vi "ATM_CLD.vi"(4 "Enter":bool, 6 "User Input":string, 7 "Card Simulator":bool, 10 "Right Buttons":T3, 11 "Left Buttons":T4) -> (0 "error out":errorcluster, 3 "ATM Messages":string, 8 "Right Menu":T1, 9 "Left Menu":T2)   [LabVIEW 2018]
doc: "ATM Version 1.0: final solution. Extensive documentation and VI appearance added"
uses:
  Controls/ATMStates.ctl
  Controls/Customer.ctl
  Controls/Messages.ctl
  <vilib>/Utility/file.llb/Read Delimited Spreadsheet (string).vi
  <vilib>/Utility/file.llb/Write Delimited Spreadsheet (string).vi
panel:
  # "CLD ATMachine v1.0"
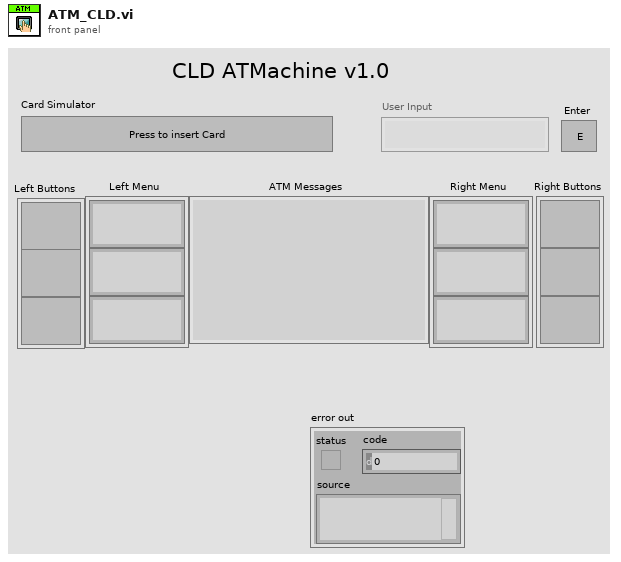
[diagram p1: front panel]
types:
  T1 = cluster{"RightString 1":string, "RightString 2":string, "RightString 3":string}
  T2 = cluster{"LeftString 1":string, "LeftString 2":string, "LeftString 3":string}
  T3 = cluster{"RightButton 1":bool, "RightButton 2":bool, "RightButton 3":bool}
  T4 = cluster{"LeftButton 1":bool, "LeftButton 2":bool, "LeftButton 3":bool}
  T5 = typedef "ATMStates.ctl" = enum16{"Initialize", "Start", "Wait for User input", "Check PIN", "Verification failed", "Wait for Menu", "Deposit", "Wait for Deposit Amount", "Deposit Complete", "Withdraw", "Wait for Withdrawal Amount", "Withdraw Complete", "Fast Cash", "Fast Cash Complete", "Withdrawal Failed", "None", "Balance Inquiry", "Return Card", "Stop"}
  T6 = typedef "Customer.ctl" = cluster{"PIN":string, "First Name":string, "Last Name":string, "Amount":string}
  T7 = typedef "Messages.ctl" = enum16{"Welcome Message", "Main Menu Message", "Account Verification Failed Message", "Session Terminate Message", "Deposit Message", "Deposit Complete Message", "Withdrawal Message", "Withdrawal Complete Message", "Withdrawal Failed Message", "Balance Inquiry Message"}
  T8 = enum8{"Enabled", "Disabled", "Disabled and Grayed Out"}
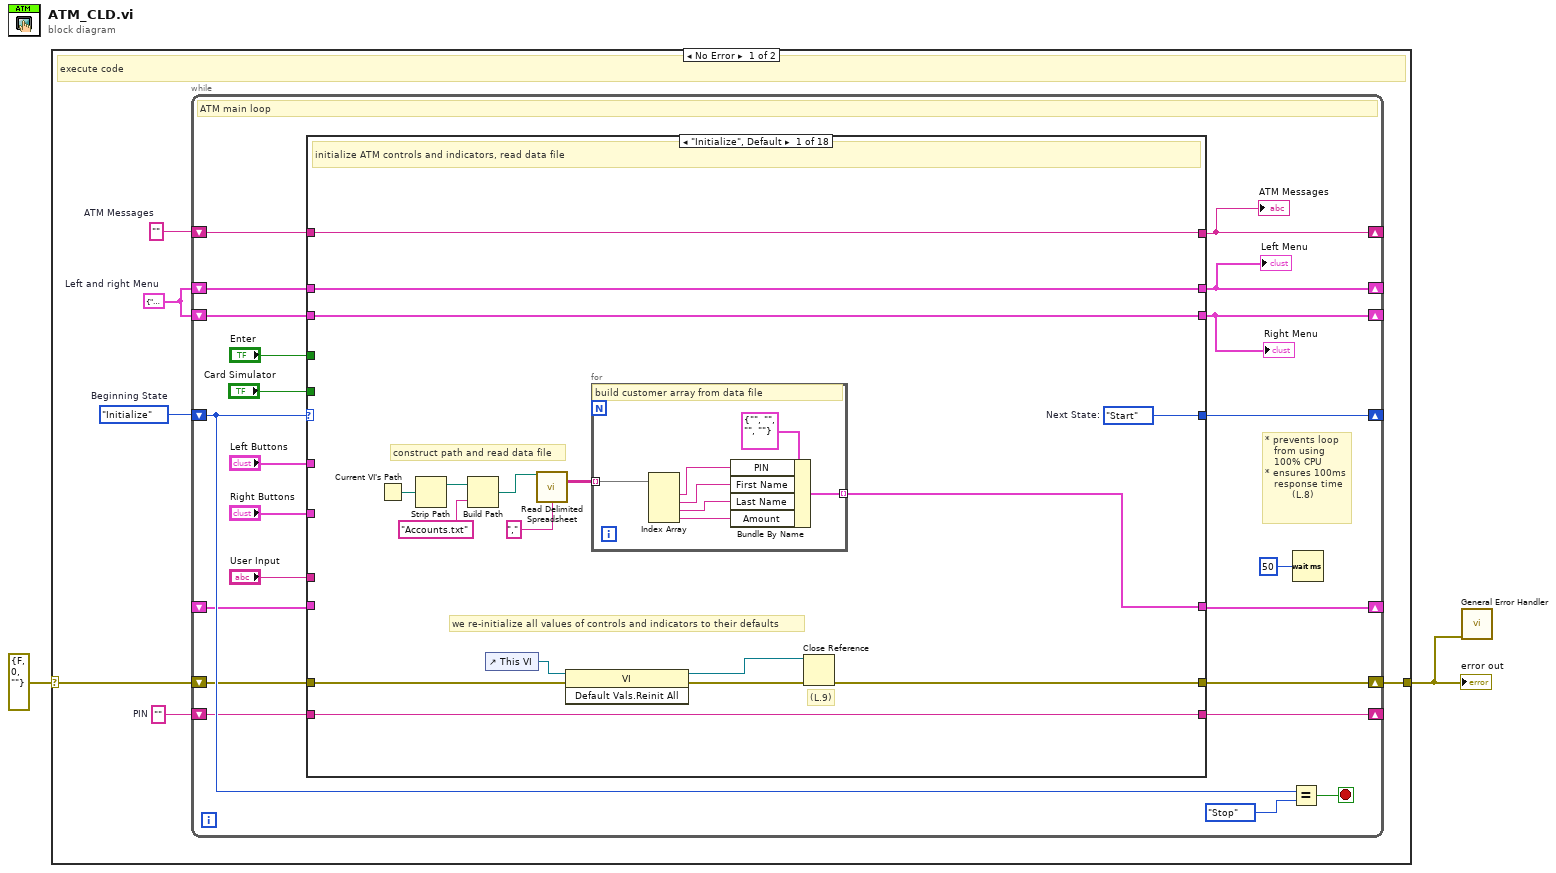
[diagram p0: block diagram]
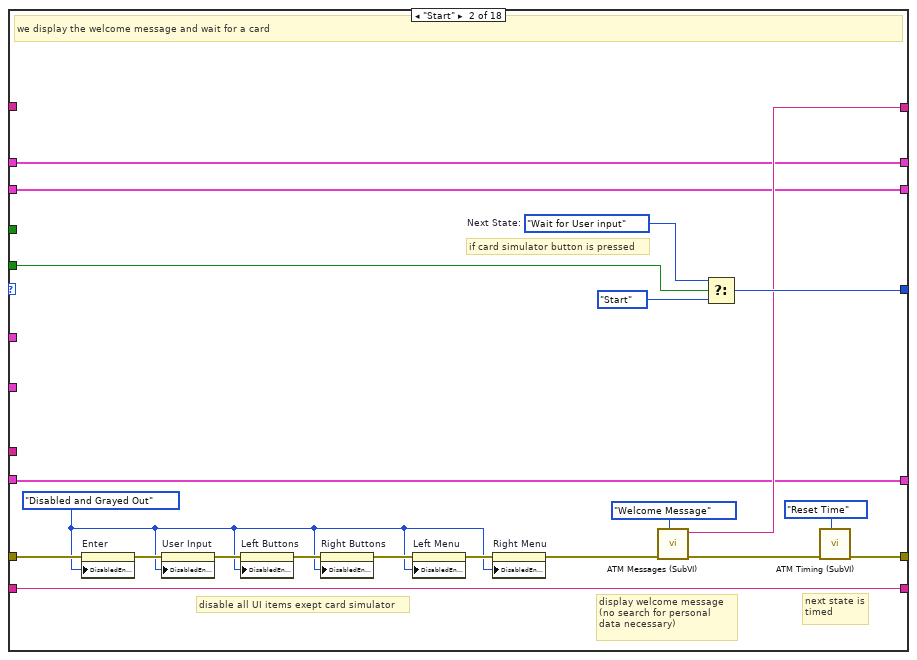
[diagram p2: hidden frame]
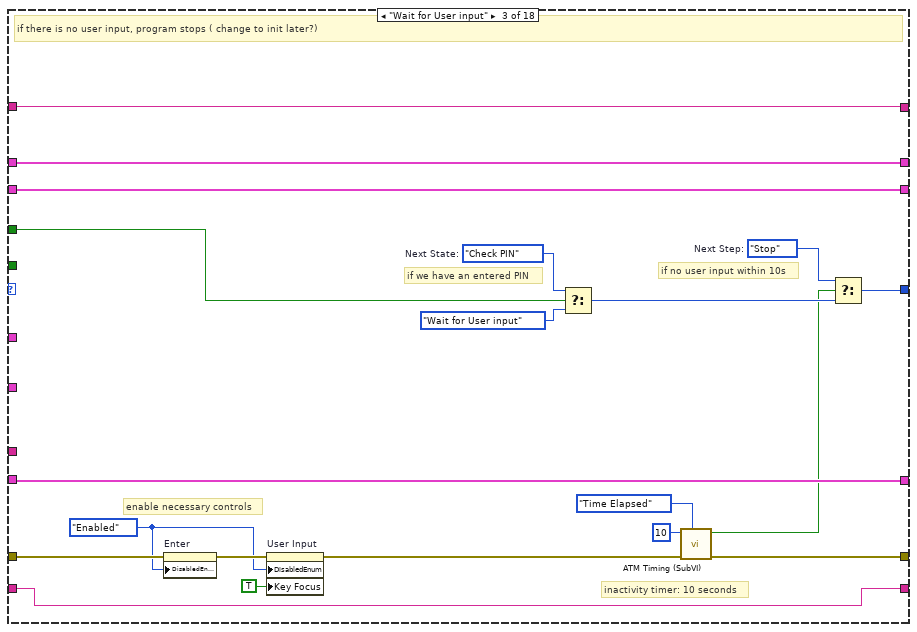
[diagram p3: hidden frame]
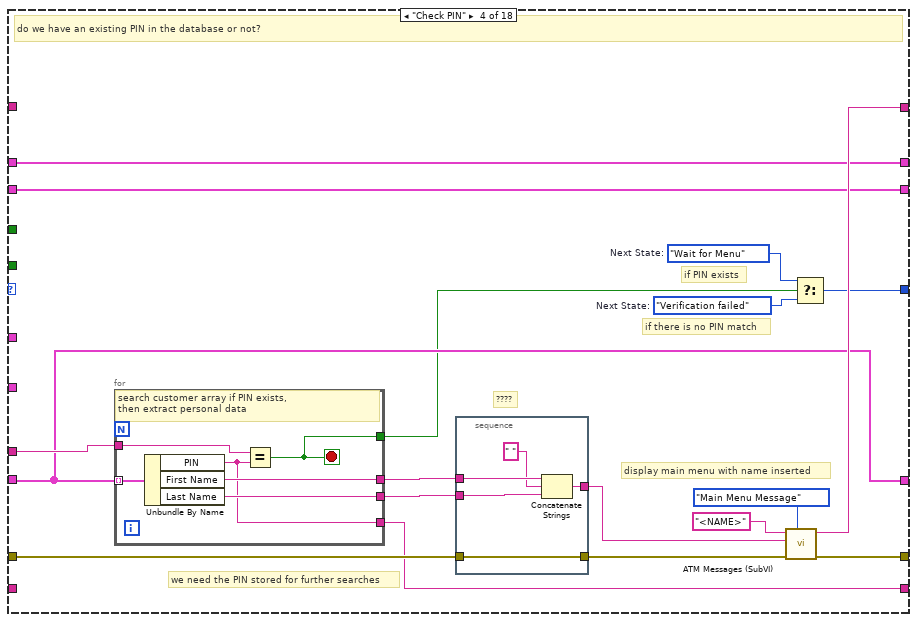
[diagram p4: hidden frame]
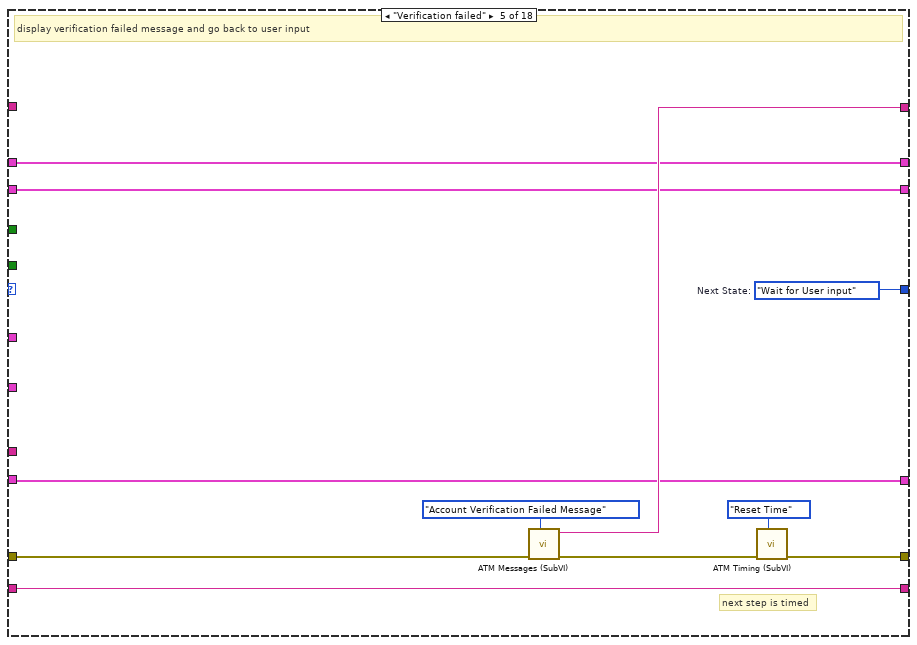
[diagram p5: hidden frame]
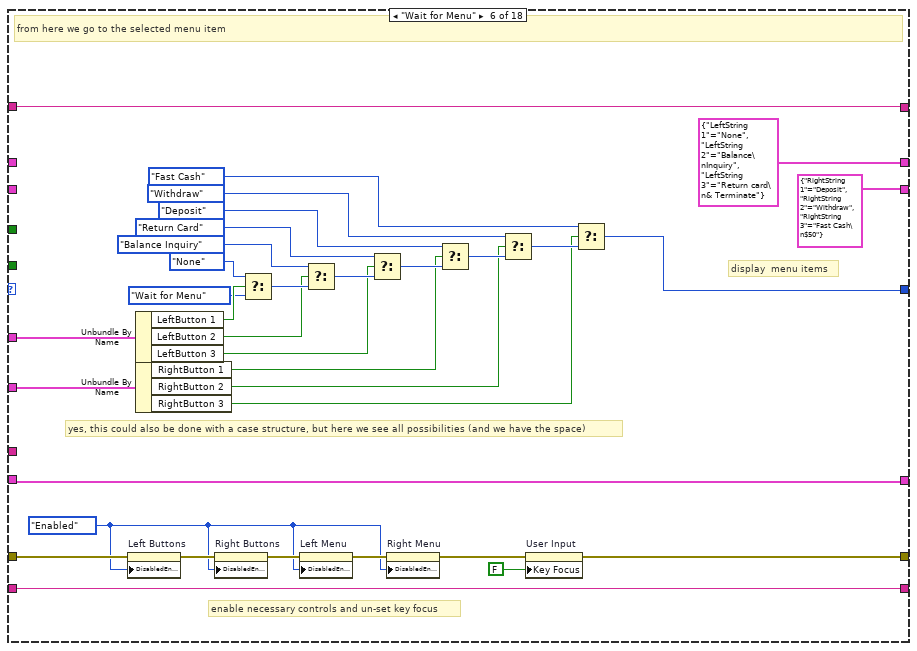
[diagram p6: hidden frame]
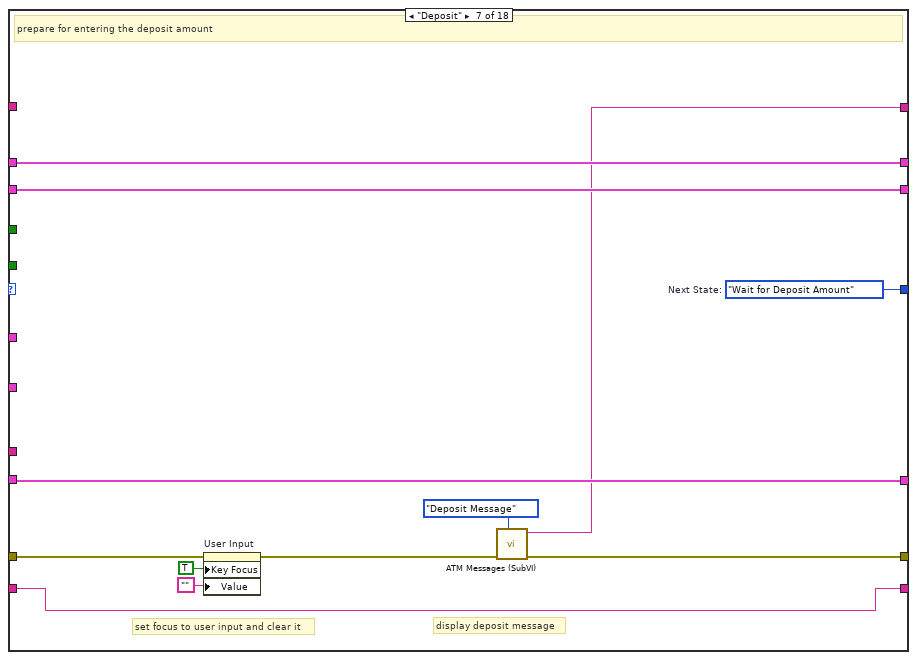
[diagram p7: hidden frame]
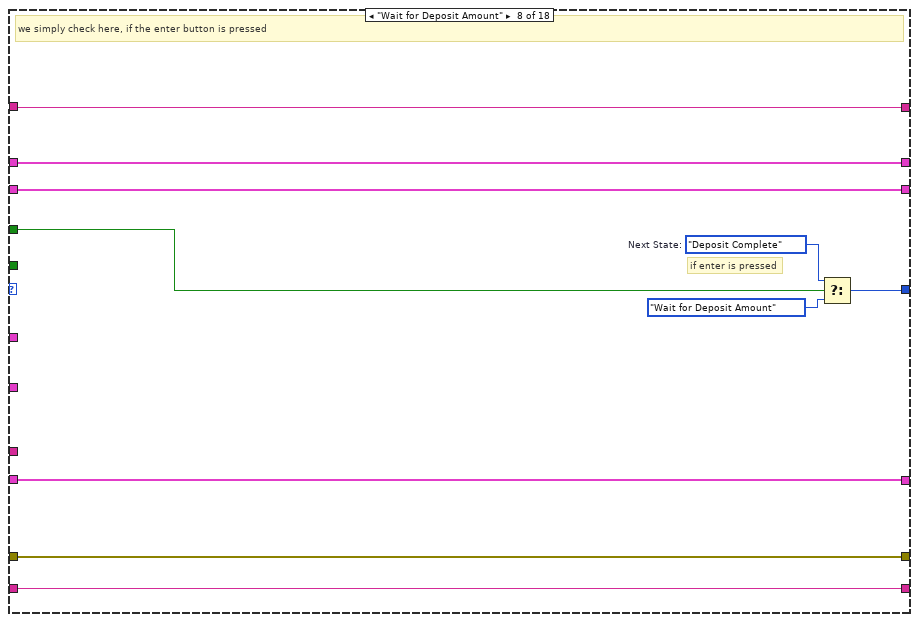
[diagram p8: hidden frame]
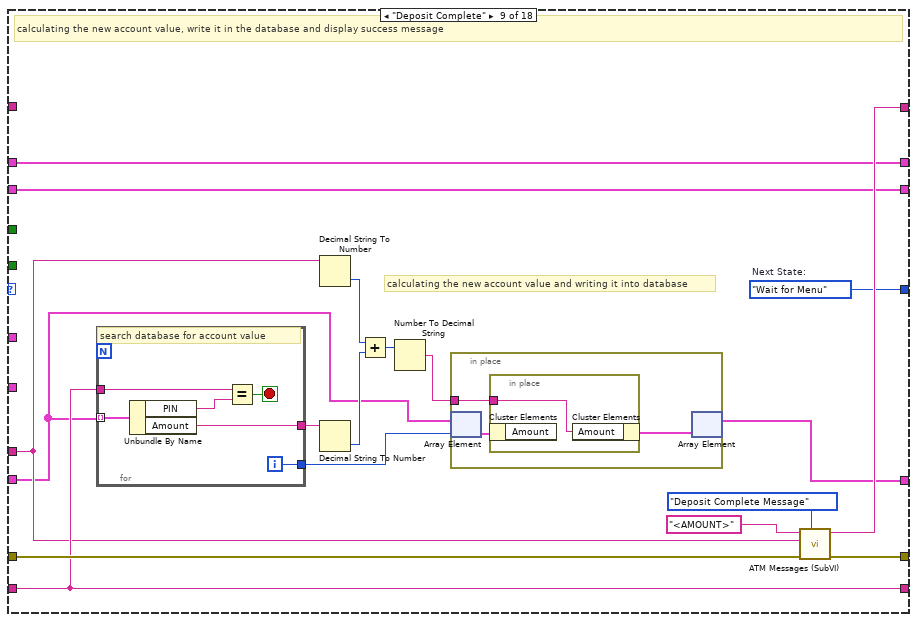
[diagram p9: hidden frame]
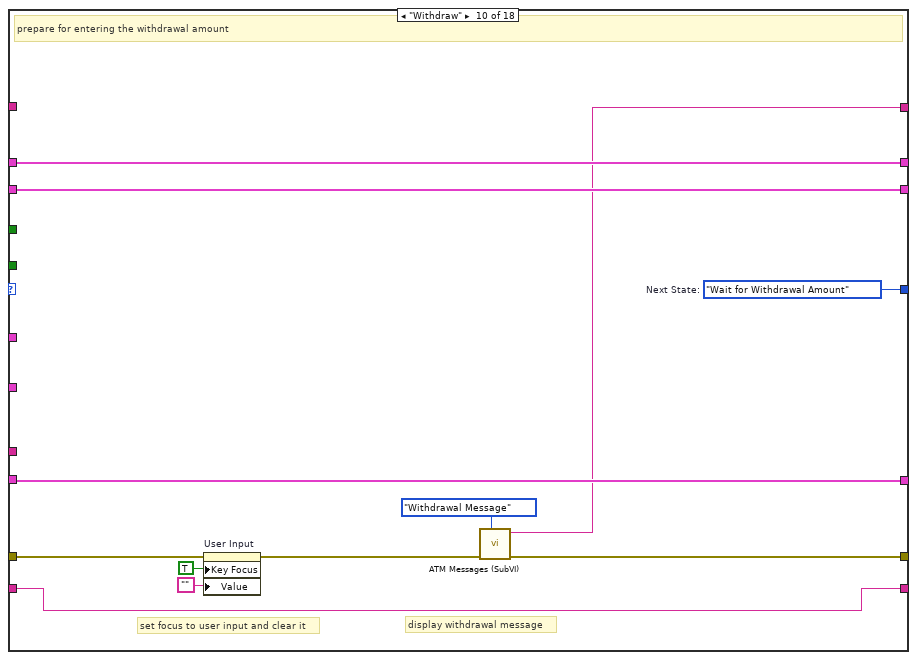
[diagram p10: hidden frame]
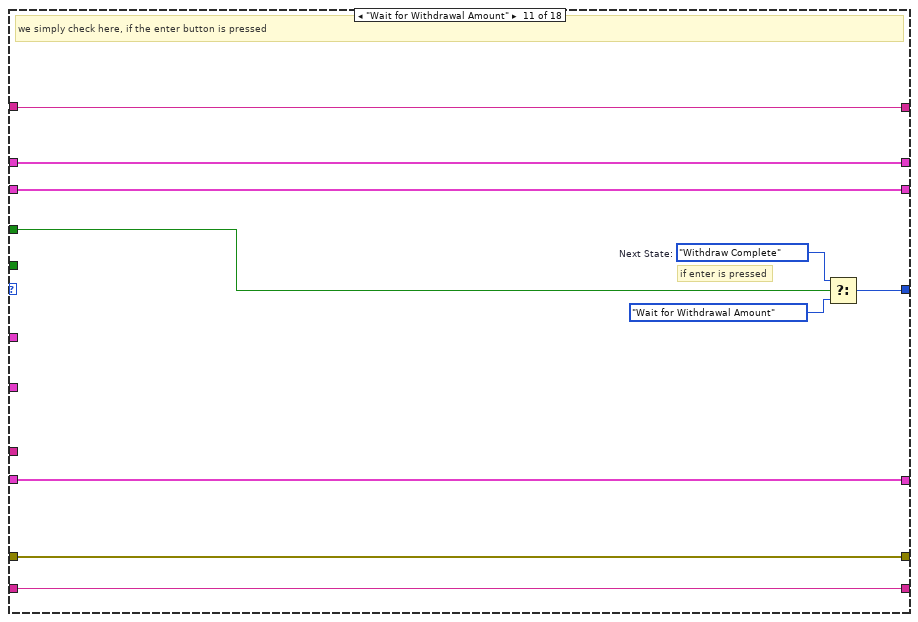
[diagram p11: hidden frame]
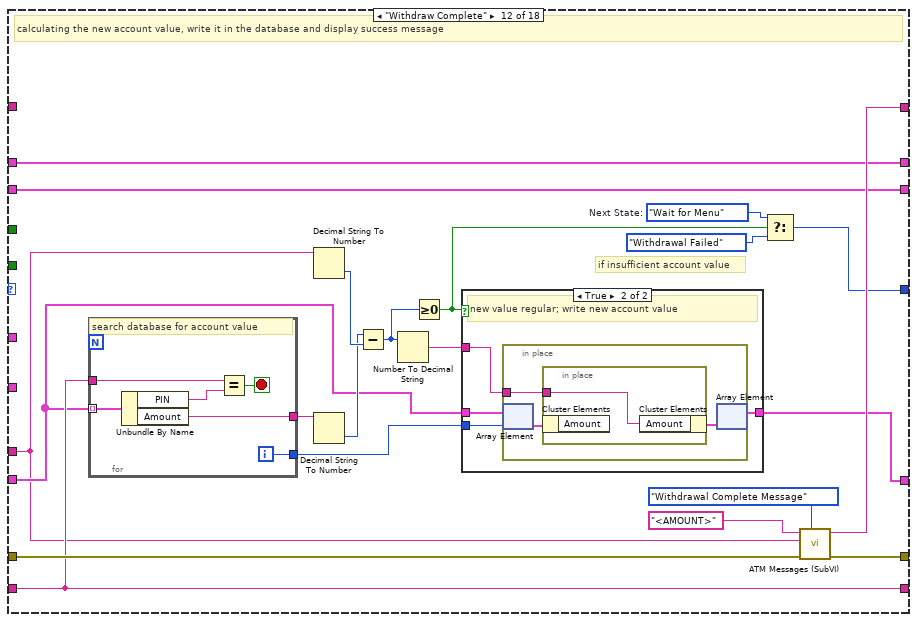
[diagram p12: hidden frame]
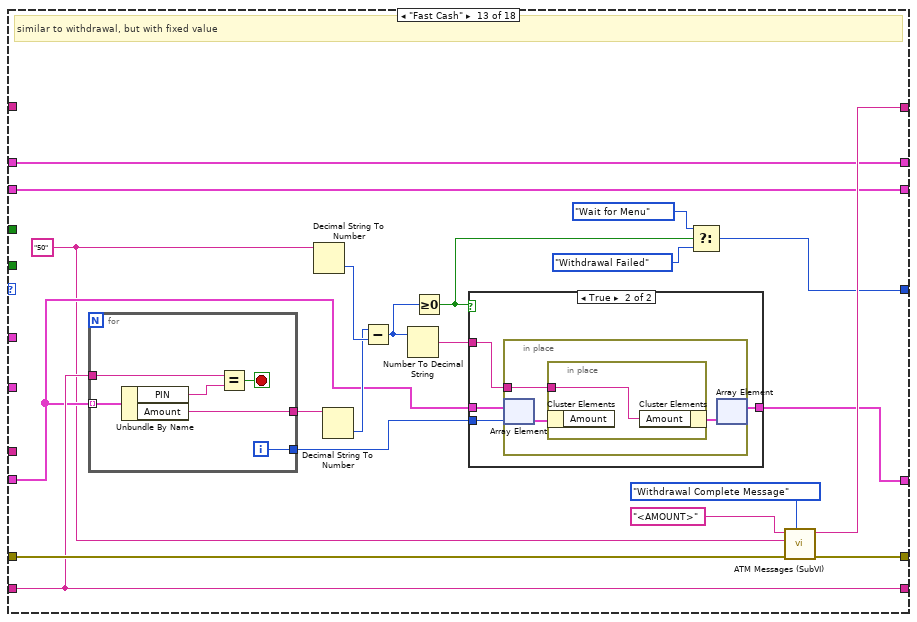
[diagram p14: hidden frame]
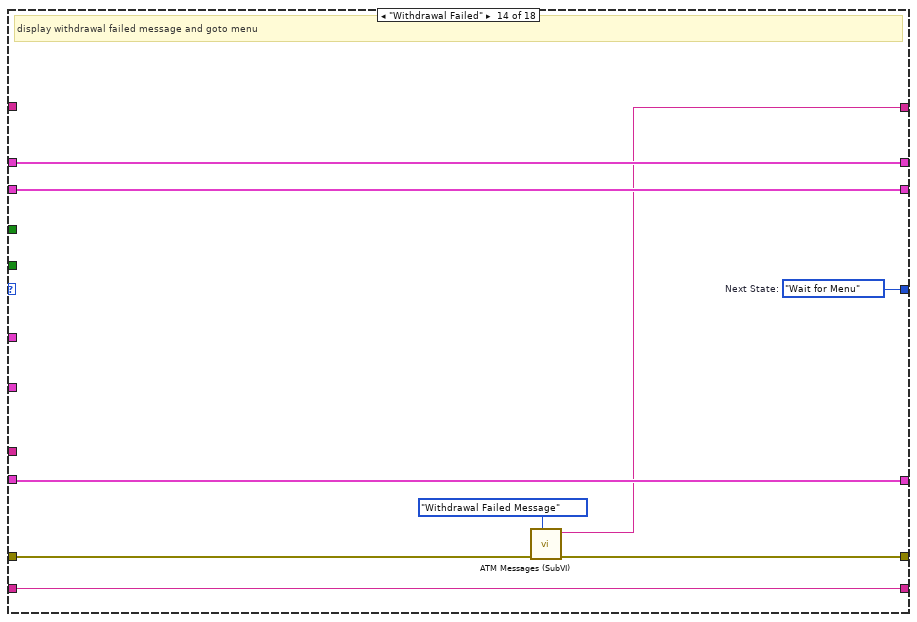
[diagram p16: hidden frame]
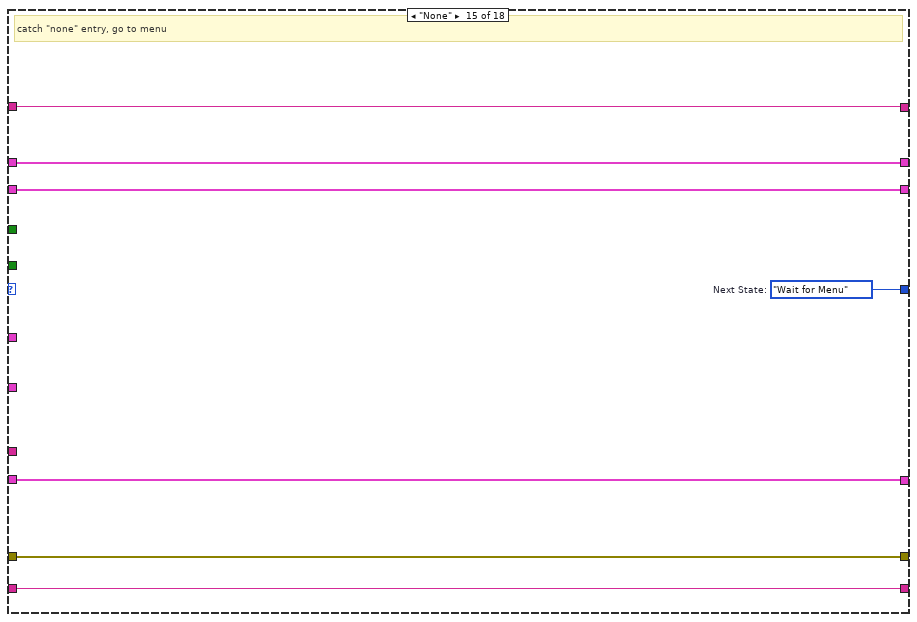
[diagram p17: hidden frame]
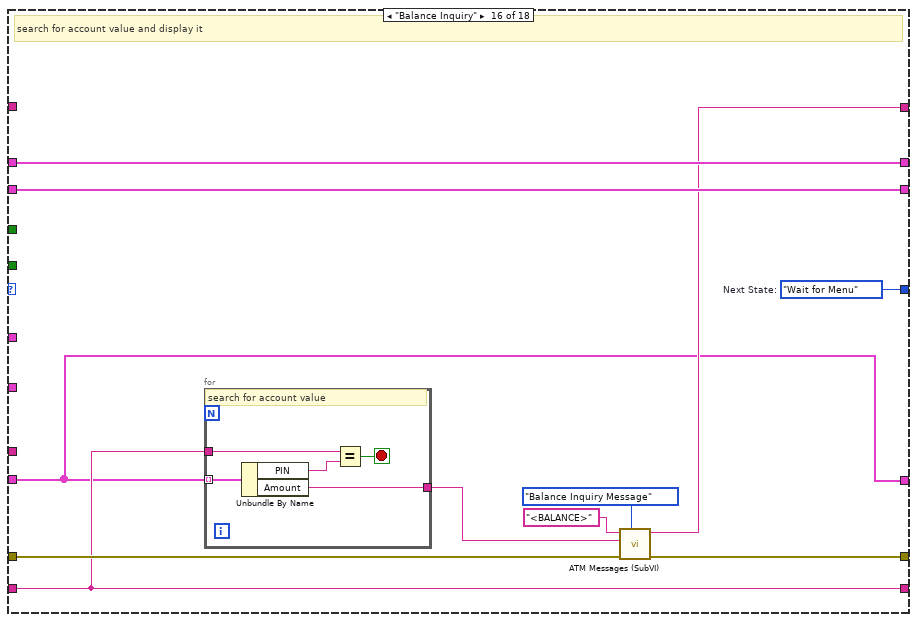
[diagram p18: hidden frame]
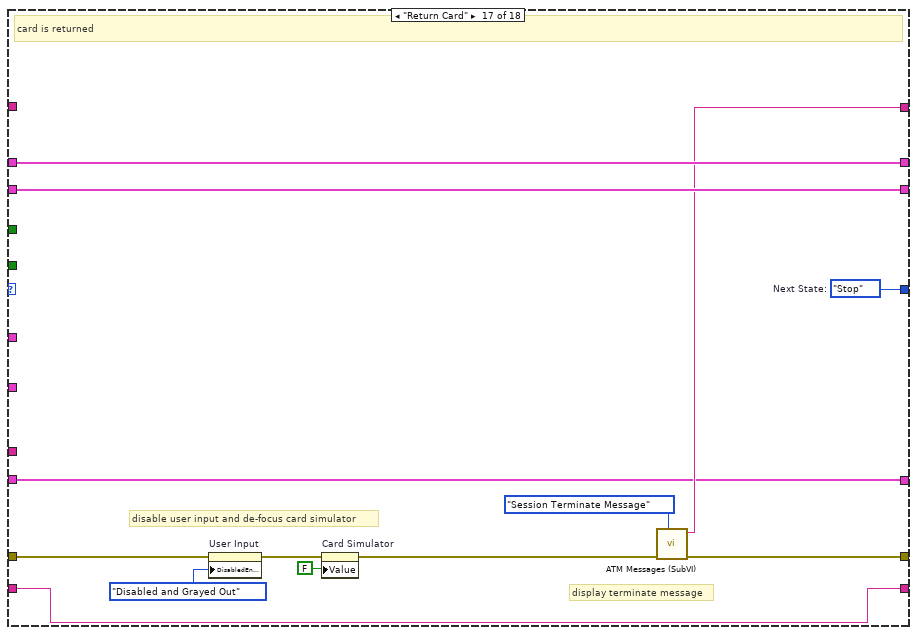
[diagram p19: hidden frame]
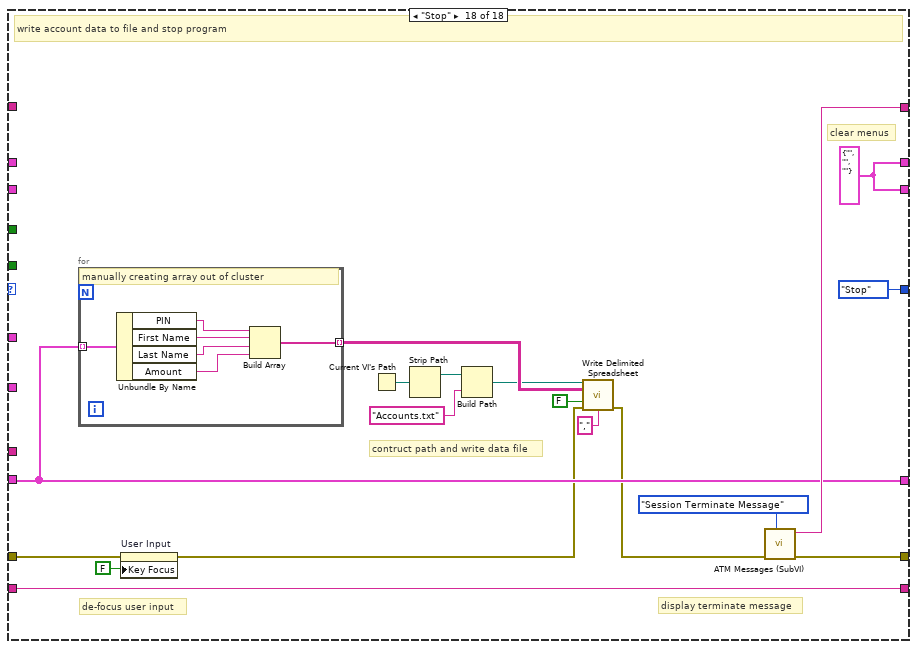
[diagram p20: hidden frame]
diagram:
  n1 = case shown="No Error" errorcluster {"status"=FALSE, "code"=0, "source"=""} ("error IO") {
    selector: errorcluster {"status"=FALSE, "code"=0, "source"=""} ("error IO") -> [w7 w383]
    tunnel: [w3 w383] -> w1
    frame No Error {
      w5 = ""  # PIN
      w4 = T2 {"LeftString 1"="", "LeftString 2"="", "LeftString 3"=""}  # Left and right Menu
      w6 = ""  # ATM Messages
      w8 = ATMStates."Initialize"  # Beginning State
      # "execute code"
      n2 = while {
        shift-right: [w27] -> _
        shift-left: w8 -> [w28]
        shift-right: [w11] -> _
        shift-left: _ -> [w24]
        shift-right: [w22] -> _
        shift-left: w6 -> [w23]
        shift-right: [w19] -> _
        shift-left: w4 -> [w17]
        shift-right: [w18] -> _
        shift-left: w4 -> [w16]
        shift-right: [w13] -> _
        shift-left: w5 -> [w12]
        shift-right: [w9] -> w3
        shift-left: w7 -> [w25]
        stop <- w30 stop-if-true
        # "* prevents loop\n   from using\n   100% CPU\n* ensures 100ms\n   response time\n         (L.8)"
        # "ATM main loop"
        n3 = case shown="\"Initialize\", Default" w28 {
          tunnel: [w42 w73 w81 w104 w135 w148 w179 w187 w203 w229 w237 w245 w282 w320 w326 w338 w347 ATMStates."Stop" ("Next State")] -> w27
          tunnel: [w43 w62 w85 w108 w130 w162 w171 w186 w206 w221 w236 w259 w295 w314 w324 w336 w348 w373] -> w9
          tunnel: w25 -> [w44 w72 w94 w98 w133 w169 w173 w186 w207 w223 w236 w260 w296 w315 w324 w335 w354 w372]
          tunnel: [w31 w57 w95 w107 w131 w159 w178 w185 w192 w228 w235 w247 w284 w319 w325 w330 w350 w369] -> w11
          tunnel: w24 -> [_ w57 w95 w107 w131 w159 w178 w185 w194 w228 w235 w249 w285 w319 w325 w330 w350 w369]
          tunnel: [w41 w65 w91 w112 w134 w158 w177 w190 w209 w227 w240 w262 w298 w317 w329 w337 w356 w375] -> w22
          tunnel: w23 -> [w41 _ w91 _ _ w158 _ w190 _ _ w240 _ _ _ w329 _ _ _]
          tunnel: "Enter" -> [_ _ w90 _ _ _ _ w191 _ _ w241 _ _ _ _ _ _ _]
          tunnel: "User Input" -> [_ _ _ w113 _ _ _ _ w199 _ _ w248 _ _ _ _ _ _]
          tunnel: [w39 w59 w78 w101 w127 T1 {"RightString 1"="Deposit", "RightString 2"="Withdraw", "RightString 3"="Fast Cash\n$50"} ("Right Menu") w180 w184 w204 w230 w234 w257 w293 w321 w327 w339 w358 w359] -> w18
          tunnel: [w40 w60 w79 w102 w128 T2 {"LeftString 1"="None", "LeftString 2"="Balance\nInquiry", "LeftString 3"="Return card\n& Terminate"} ("Left Menu") w181 w183 w205 w231 w233 w258 w294 w322 w328 w340 w357 w359] -> w19
          tunnel: w17 -> [w40 w60 w79 w102 w128 _ w181 w183 w205 w231 w233 w258 w294 w322 w328 w340 w357 _]
          tunnel: w16 -> [w39 w59 w78 w101 w127 _ w180 w184 w204 w230 w234 w257 w293 w321 w327 w339 w358 _]
          tunnel: "Left Buttons" -> [_ _ _ _ _ w136 _ _ _ _ _ _ _ _ _ _ _ _]
          tunnel: "Right Buttons" -> [_ _ _ _ _ w157 _ _ _ _ _ _ _ _ _ _ _ _]
          tunnel: [w38 w58 w77 w96 w126 w137 w170 w182 w201 w220 w232 w255 w291 w318 w323 w332 w346 w370] -> w13
          tunnel: w12 -> [w38 w58 w77 _ w126 w137 w170 w182 w201 w220 w232 w255 w291 w318 w323 w332 w346 w370]
          tunnel: "Card Simulator" -> [_ w55 _ _ _ _ _ _ _ _ _ _ _ _ _ _ _ _]
          frame "Initialize", Default {
            w42 = ATMStates."Start"  # Next State:
            # "construct path and read data file"
            # "(L.9)"
            # "we re-initialize all values of controls and indicators to their defaults"
            # "initialize ATM controls and indicators, read data file"
            n4 = Current VI's Path() -> (path=w37:path)
            n5 = Strip Path(path=w37) -> (stripped path=w36:path)  [unwired: 1 out]
            n6 = Build Path(base path=w36, name or relative path="Accounts.txt") -> (appended path=w35:path)
            n7 = control-ref of="This VI"() -> (w47:refnum<vi>)
            n8 = call-poly <vilib>:"Read Delimited Spreadsheet.vi"("file path (dialog if empty)"=w35, "delimiter (\\t)"="," ("delimiter (\\t)")) -> ("all rows"=w32:string[][])  [unwired: 8 in, 5 out]
            n9 = invoke class="VI" method="Default Vals.Reinit All"(reference=w47, error in=w44) -> (reference out=w46:refnum<vi>, error out=w45:errorcluster)  [unwired: 1 in, 1 out]
            n10 = for {
              tunnel: w32 -> [w54] mode=indexing
              tunnel: [w52] -> w31 mode=indexing
              # "build customer array from data file"
              n11 = Index Array(array=w54) -> (element #1=w51:string, element #2=w50:string, element #3=w49:string, element #4=w48:string)  [unwired: 4 in]
              n12 = Bundle By Name(cluster=T6 {"PIN"="", "First Name"="", "Last Name"="", "Amount"=""} ("Cluster"), "PIN"=w51, "First Name"=w50, "Last Name"=w49, "Amount"=w48) -> (w52:T6)
            }
            n13 = Close Reference(reference=w46, error in (no error)=w45) -> (error out=w43:errorcluster)
          }
          frame "Start" {
            w66 = T8."Disabled and Grayed Out" ("Disabled")
            w75 = ATMStates."Wait for User input"  # Next State:
            # "next state is\ntimed"
            # "if card simulator button is pressed"
            # "display welcome message\n(no search for personal \ndata necessary)"
            # "disable all UI items exept card simulator"
            # "we display the welcome message and wait for a card"
            n14 = property on="Enter" class="Bool"(error in=w72, "DisabledEnum"=w66) -> (error out=w71:errorcluster)  [unwired: 1 in, 1 out]
            n15 = property on="User Input" class="Str"(error in=w71, "DisabledEnum"=w66) -> (error out=w70:errorcluster)  [unwired: 1 in, 1 out]
            n16 = property on="Left Buttons" class="Clust"(error in=w70, "DisabledEnum"=w66) -> (error out=w69:errorcluster)  [unwired: 1 in, 1 out]
            n17 = property on="Right Buttons" class="Clust"(error in=w69, "DisabledEnum"=w66) -> (error out=w68:errorcluster)  [unwired: 1 in, 1 out]
            n18 = property on="Left Menu" class="Clust (strict)"(error in=w68, "DisabledEnum"=w66) -> (error out=w67:errorcluster)  [unwired: 1 in, 1 out]
            n19 = property on="Right Menu" class="Clust (strict)"(error in=w67, "DisabledEnum"=w66) -> (error out=w63:errorcluster)  [unwired: 1 in, 1 out]
            n20 = call "ATM Messages (SubVI).vi"("Message Type"=Messages."Welcome Message", "error in (no error)"=w63) -> ("error out"=w61:errorcluster, "Message out"=w65:string)  [unwired: 8 in]
            n21 = Select(t=w75, s=w55, f=ATMStates."Start" ("Next State")) -> (s? t:f=w73:T5)
            n22 = call "ATM Timing (SubVI).vi"("Function"=enum16{"Reset Time", "Time Elapsed"}."Reset Time", "error in (no error)"=w61) -> ("error out"=w62:errorcluster)  [unwired: 7 in, 2 out]
          }
          frame "Wait for User input" {
            w80 = ATMStates."Stop"  # Next Step:
            w88 = ATMStates."Check PIN"  # Next State:
            w92 = T8."Enabled" ("Disabled")
            # "if we have an entered PIN"
            # "if no user input within 10s"
            # "inactivity timer: 10 seconds"
            # "enable necessary controls"
            # "if there is no user input, program stops ( change to init later?)"
            n23 = property on="Enter" class="Bool"(error in=w94, "DisabledEnum"=w92) -> (error out=w93:errorcluster)  [unwired: 1 in, 1 out]
            n24 = property on="User Input" class="Str"(error in=w93, "DisabledEnum"=w92, "Key Focus"=TRUE) -> (error out=w86:errorcluster)  [unwired: 1 in, 1 out]
            n25 = Select(t=w88, s=w90, f=ATMStates."Wait for User input" ("Next State")) -> (s? t:f=w83:T5)
            n26 = call "ATM Timing (SubVI).vi"("Function"=enum16{"Reset Time", "Time Elapsed"}."Time Elapsed", "error in (no error)"=w86, "Time to Wait (s)"=10) -> ("error out"=w85:errorcluster, "Time elapsed ?"=w82:bool)  [unwired: 6 in, 1 out]
            n27 = Select(t=w80, s=w82, f=w83) -> (s? t:f=w81:T5)
          }
          frame "Check PIN" {
            w103 = ATMStates."Verification failed"  # Next State:
            w105 = ATMStates."Wait for Menu"  # Next State:
            # "if there is no PIN match"
            # "if PIN exists"
            # "display main menu with name inserted"
            # "we need the PIN stored for further searches"
            # "????"
            # "do we have an existing PIN in the database or not?"
            n28 = for {
              tunnel: w107 -> [w124] mode=indexing
              tunnel: [w123] -> w109
              tunnel: [w122] -> w106
              tunnel: w113 -> [w121]
              tunnel: [w120] -> w99
              tunnel: [w119] -> w96
              stop <- w120 stop-if-true
              # "search customer array if PIN exists,\nthen extract personal data"
              n29 = Unbundle By Name(w124) -> ("PIN"=w119:string, "First Name"=w123:string, "Last Name"=w122:string)
              n30 = Equal?(x=w121, y=w119) -> (x = y?=w120:bool)
            }
            n31 = stacked-sequence {
              tunnel: w109 -> [w118]
              tunnel: w106 -> [w116]
              tunnel: [w115] -> w100
              tunnel: w98 -> [w114]
              tunnel: [w114] -> w97
              frame #0 {
                n32 = Concatenate Strings(w118, " " ("string"), w116) -> (w115:string)
              }
            }
            n33 = call "ATM Messages (SubVI).vi"("Message Type"=Messages."Main Menu Message", "error in (no error)"=w97, "replace string (\"\")"=w100, "search string"="<NAME>") -> ("error out"=w108:errorcluster, "Message out"=w112:string)  [unwired: 6 in]
            n34 = Select(t=w105, s=w99, f=w103) -> (s? t:f=w104:T5)
          }
          frame "Verification failed" {
            w135 = ATMStates."Wait for User input"  # Next State:
            # "next step is timed"
            # "display verification failed message and go back to user input"
            n35 = call "ATM Messages (SubVI).vi"("Message Type"=Messages."Account Verification Failed Message", "error in (no error)"=w133) -> ("error out"=w129:errorcluster, "Message out"=w134:string)  [unwired: 8 in]
            n36 = call "ATM Timing (SubVI).vi"("Function"=enum16{"Reset Time", "Time Elapsed"}."Reset Time", "error in (no error)"=w129) -> ("error out"=w130:errorcluster)  [unwired: 7 in, 2 out]
          }
          frame "Wait for Menu" {
            w165 = T8."Enabled" ("Disabled")
            # "display  menu items"
            # "enable necessary controls and un-set key focus"
            # "yes, this could also be done with a case structure, but here we see all possibilities (and we have the space)"
            # "from here we go to the selected menu item"
            n37 = property on="Left Buttons" class="Clust"(error in=w169, "DisabledEnum"=w165) -> (error out=w168:errorcluster)  [unwired: 1 in, 1 out]
            n38 = Unbundle By Name(w136) -> ("LeftButton 1"=w155:bool, "LeftButton 2"=w147:bool, "LeftButton 3"=w146:bool)
            n39 = Unbundle By Name(w157) -> ("RightButton 1"=w145:bool, "RightButton 2"=w144:bool, "RightButton 3"=w143:bool)
            n40 = property on="Right Buttons" class="Clust"(error in=w168, "DisabledEnum"=w165) -> (error out=w167:errorcluster)  [unwired: 1 in, 1 out]
            n41 = Select(t=ATMStates."None" ("Next State"), s=w155, f=ATMStates."Wait for Menu" ("Next State")) -> (s? t:f=w154:T5)
            n42 = property on="Left Menu" class="Clust (strict)"(error in=w167, "DisabledEnum"=w165) -> (error out=w166:errorcluster)  [unwired: 1 in, 1 out]
            n43 = Select(t=ATMStates."Balance Inquiry", s=w147, f=w154) -> (s? t:f=w152:T5)
            n44 = Select(t=ATMStates."Return Card", s=w146, f=w152) -> (s? t:f=w151:T5)
            n45 = property on="Right Menu" class="Clust (strict)"(error in=w166, "DisabledEnum"=w165) -> (error out=w164:errorcluster)  [unwired: 1 in, 1 out]
            n46 = Select(t=ATMStates."Deposit", s=w145, f=w151) -> (s? t:f=w150:T5)
            n47 = Select(t=ATMStates."Withdraw", s=w144, f=w150) -> (s? t:f=w149:T5)
            n48 = property on="User Input" class="Str"(error in=w164, "Key Focus"=FALSE) -> (error out=w162:errorcluster)  [unwired: 1 in, 1 out]
            n49 = Select(t=ATMStates."Fast Cash", s=w143, f=w149) -> (s? t:f=w148:T5)
          }
          frame "Deposit" {
            w179 = ATMStates."Wait for Deposit Amount"  # Next State:
            # "display deposit message"
            # "set focus to user input and clear it"
            # "prepare for entering the deposit amount"
            n50 = property on="User Input" class="Str"(error in=w173, "Key Focus"=TRUE, "Value"="") -> (error out=w172:errorcluster)  [unwired: 1 in, 1 out]
            n51 = call "ATM Messages (SubVI).vi"("Message Type"=Messages."Deposit Message", "error in (no error)"=w172) -> ("error out"=w171:errorcluster, "Message out"=w177:string)  [unwired: 8 in]
          }
          frame "Wait for Deposit Amount" {
            w189 = ATMStates."Deposit Complete"  # Next State:
            # "if enter is pressed"
            # "we simply check here, if the enter button is pressed"
            n52 = Select(t=w189, s=w191, f=ATMStates."Wait for Deposit Amount" ("Next State")) -> (s? t:f=w187:T5)
          }
          frame "Deposit Complete" {
            w203 = ATMStates."Wait for Menu"  # Next State:
            # "calculating the new account value and writing it into database"
            # "calculating the new account value, write it in the database and display success message"
            n53 = for {
              tunnel: w194 -> [w219] mode=indexing
              tunnel: [w217] -> w200
              tunnel: w201 -> [w216]
              tunnel: [w214] -> w195
              i -> [w214]
              stop <- w215 stop-if-true
              # "search database for account value"
              n54 = Unbundle By Name(w219) -> ("PIN"=w218:string, "Amount"=w217:string)
              n55 = Equal?(x=w216, y=w218) -> (x = y?=w215:bool)
            }
            n56 = Decimal String To Number(string=w199) -> (number=w198:i32)  [unwired: 2 in, 1 out]
            n57 = Decimal String To Number(string=w200) -> (number=w197:i32)  [unwired: 2 in, 1 out]
            n58 = Add(x=w198, y=w197) -> (x+y=w196:i32)
            n59 = Number To Decimal String(number=w196) -> (decimal integer string=w193:string)  [unwired: 1 in]
            n60 = in-place {
              in-place-border: w193 -> [w210]
              n61 = in-place-array #1(w194, w195) -> (w212:T6)
              n62 = in-place {
                in-place-border: w210 -> [w213]
                n63 = in-place-cluster #2(w212) -> ()  [unwired: 1 out]
                n64 = in-place-cluster #2("Amount"=w213) -> (w211:T6)
              }
              n65 = in-place-array #1(w211) -> (w192:T6[])  [unwired: 1 out]
            }
            n66 = call "ATM Messages (SubVI).vi"("Message Type"=Messages."Deposit Complete Message", "error in (no error)"=w207, "replace string (\"\")"=w199, "search string"="<AMOUNT>") -> ("error out"=w206:errorcluster, "Message out"=w209:string)  [unwired: 6 in]
          }
          frame "Withdraw" {
            w229 = ATMStates."Wait for Withdrawal Amount"  # Next State:
            # "display withdrawal message"
            # "set focus to user input and clear it"
            # "prepare for entering the withdrawal amount"
            n67 = property on="User Input" class="Str"(error in=w223, "Key Focus"=TRUE, "Value"="") -> (error out=w222:errorcluster)  [unwired: 1 in, 1 out]
            n68 = call "ATM Messages (SubVI).vi"("Message Type"=Messages."Withdrawal Message", "error in (no error)"=w222) -> ("error out"=w221:errorcluster, "Message out"=w227:string)  [unwired: 8 in]
          }
          frame "Wait for Withdrawal Amount" {
            w239 = ATMStates."Withdraw Complete"  # Next State:
            # "if enter is pressed"
            # "we simply check here, if the enter button is pressed"
            n69 = Select(t=w239, s=w241, f=ATMStates."Wait for Withdrawal Amount" ("Next State")) -> (s? t:f=w237:T5)
          }
          frame "Withdraw Complete" {
            w244 = ATMStates."Wait for Menu"  # Next State:
            # "if insufficient account value"
            # "calculating the new account value, write it in the database and display success message"
            n70 = for {
              tunnel: w249 -> [w277] mode=indexing
              tunnel: [w275] -> w250
              tunnel: w255 -> [w274]
              tunnel: [w272] -> w251
              i -> [w272]
              stop <- w273 stop-if-true
              # "search database for account value"
              n71 = Unbundle By Name(w277) -> ("PIN"=w276:string, "Amount"=w275:string)
              n72 = Equal?(x=w274, y=w276) -> (x = y?=w273:bool)
            }
            n73 = Decimal String To Number(string=w248) -> (number=w254:i32)  [unwired: 2 in, 1 out]
            n74 = Decimal String To Number(string=w250) -> (number=w253:i32)  [unwired: 2 in, 1 out]
            n75 = Subtract(x=w253, y=w254) -> (x-y=w246:i32)
            n76 = Number To Decimal String(number=w246) -> (decimal integer string=w252:string)  [unwired: 1 in]
            n77 = Greater Or Equal To 0?(x=w246) -> (x >= 0?=w243:bool)
            n78 = case shown="True" w243 {
              tunnel: w252 -> [_ w267]
              tunnel: w251 -> [_ w266]
              tunnel: w249 -> [w263 w265]
              tunnel: [w263 w264] -> w247
              frame False {
              }
              frame True {
                # "new value regular; write new account value"
                n79 = in-place {
                  in-place-border: w267 -> [w268]
                  n80 = in-place-array #3(w265, w266) -> (w270:T6)
                  n81 = in-place {
                    in-place-border: w268 -> [w271]
                    n82 = in-place-cluster #4(w270) -> ()  [unwired: 1 out]
                    n83 = in-place-cluster #4("Amount"=w271) -> (w269:T6)
                  }
                  n84 = in-place-array #3(w269) -> (w264:T6[])  [unwired: 1 out]
                }
              }
            }
            n85 = Select(t=w244, s=w243, f=ATMStates."Withdrawal Failed" ("Next State")) -> (s? t:f=w245:T5)
            n86 = call "ATM Messages (SubVI).vi"("Message Type"=Messages."Withdrawal Complete Message", "error in (no error)"=w260, "replace string (\"\")"=w248, "search string"="<AMOUNT>") -> ("error out"=w259:errorcluster, "Message out"=w262:string)  [unwired: 6 in]
          }
          frame "Fast Cash" {
            w278 = "50"
            # "similar to withdrawal, but with fixed value"
            n87 = for {
              tunnel: w285 -> [w313] mode=indexing
              tunnel: [w311] -> w286
              tunnel: w291 -> [w310]
              tunnel: [w308] -> w287
              i -> [w308]
              stop <- w309 stop-if-true
              n88 = Unbundle By Name(w313) -> ("PIN"=w312:string, "Amount"=w311:string)
              n89 = Equal?(x=w310, y=w312) -> (x = y?=w309:bool)
            }
            n90 = Decimal String To Number(string=w278) -> (number=w290:i32)  [unwired: 2 in, 1 out]
            n91 = Decimal String To Number(string=w286) -> (number=w289:i32)  [unwired: 2 in, 1 out]
            n92 = Subtract(x=w289, y=w290) -> (x-y=w283:i32)
            n93 = Number To Decimal String(number=w283) -> (decimal integer string=w288:string)  [unwired: 1 in]
            n94 = Greater Or Equal To 0?(x=w283) -> (x >= 0?=w280:bool)
            n95 = case shown="True" w280 {
              tunnel: w288 -> [_ w303]
              tunnel: w287 -> [_ w302]
              tunnel: w285 -> [w299 w301]
              tunnel: [w299 w300] -> w284
              frame False {
              }
              frame True {
                n96 = in-place {
                  in-place-border: w303 -> [w304]
                  n97 = in-place-array #5(w301, w302) -> (w306:T6)
                  n98 = in-place {
                    in-place-border: w304 -> [w307]
                    n99 = in-place-cluster #6(w306) -> ()  [unwired: 1 out]
                    n100 = in-place-cluster #6("Amount"=w307) -> (w305:T6)
                  }
                  n101 = in-place-array #5(w305) -> (w300:T6[])  [unwired: 1 out]
                }
              }
            }
            n102 = Select(t=ATMStates."Wait for Menu" ("Next State"), s=w280, f=ATMStates."Withdrawal Failed" ("Next State")) -> (s? t:f=w282:T5)
            n103 = call "ATM Messages (SubVI).vi"("Message Type"=Messages."Withdrawal Complete Message", "error in (no error)"=w296, "replace string (\"\")"=w278, "search string"="<AMOUNT>") -> ("error out"=w295:errorcluster, "Message out"=w298:string)  [unwired: 6 in]
          }
          frame "Withdrawal Failed" {
            w320 = ATMStates."Wait for Menu"  # Next State:
            # "display withdrawal failed message and goto menu"
            n104 = call "ATM Messages (SubVI).vi"("Message Type"=Messages."Withdrawal Failed Message", "error in (no error)"=w315) -> ("error out"=w314:errorcluster, "Message out"=w317:string)  [unwired: 8 in]
          }
          frame "None" {
            w326 = ATMStates."Wait for Menu"  # Next State:
            # "catch \"none\" entry, go to menu"
          }
          frame "Balance Inquiry" {
            w338 = ATMStates."Wait for Menu"  # Next State:
            # "search for account value and display it"
            n105 = for {
              tunnel: w330 -> [w345] mode=indexing
              tunnel: [w343] -> w331
              tunnel: w332 -> [w342]
              stop <- w341 stop-if-true
              # "search for account value"
              n106 = Unbundle By Name(w345) -> ("PIN"=w344:string, "Amount"=w343:string)
              n107 = Equal?(x=w342, y=w344) -> (x = y?=w341:bool)
            }
            n108 = call "ATM Messages (SubVI).vi"("Message Type"=Messages."Balance Inquiry Message", "error in (no error)"=w335, "replace string (\"\")"=w331, "search string"="<BALANCE>") -> ("error out"=w336:errorcluster, "Message out"=w337:string)  [unwired: 6 in]
          }
          frame "Return Card" {
            w347 = ATMStates."Stop"  # Next State:
            # "display terminate message"
            # "disable user input and de-focus card simulator"
            # "card is returned"
            n109 = property on="User Input" class="Str"(error in=w354, "DisabledEnum"=T8."Disabled and Grayed Out" ("Disabled")) -> (error out=w353:errorcluster)  [unwired: 1 in, 1 out]
            n110 = property on="Card Simulator" class="Bool (strict)"(error in=w353, "Value"=FALSE ("Card Simulator")) -> (error out=w349:errorcluster)  [unwired: 1 in, 1 out]
            n111 = call "ATM Messages (SubVI).vi"("Message Type"=Messages."Session Terminate Message", "error in (no error)"=w349) -> ("error out"=w348:errorcluster, "Message out"=w356:string)  [unwired: 8 in]
          }
          frame "Stop" {
            w359 = T2 {"LeftString 1"="", "LeftString 2"="", "LeftString 3"=""} ("Left Menu")
            # "display terminate message"
            # "clear menus"
            # "de-focus user input"
            # "contruct path and write data file"
            # "write account data to file and stop program"
            n112 = for {
              tunnel: w369 -> [w382] mode=indexing
              tunnel: [w377] -> w365 mode=indexing
              # "manually creating array out of cluster"
              n113 = Unbundle By Name(w382) -> ("PIN"=w381:string, "First Name"=w380:string, "Last Name"=w379:string, "Amount"=w378:string)
              n114 = Build Array "Build Array"(w381, w380, w379, w378) -> (w377:string[])
            }
            n115 = property on="User Input" class="Str"(error in=w372, "Key Focus"=FALSE) -> (error out=w361:errorcluster)  [unwired: 1 in, 1 out]
            n116 = Current VI's Path() -> (path=w368:path)
            n117 = Strip Path(path=w368) -> (stripped path=w367:path)  [unwired: 1 out]
            n118 = Build Path(base path=w367, name or relative path="Accounts.txt") -> (appended path=w364:path)
            n119 = call-poly <vilib>:"Write Delimited Spreadsheet.vi"("file path (dialog if empty)"=w364, "2D data"=w365, "append to file? (new file:F)"=FALSE, "error in (no error)"=w361, "delimiter (\\t)"="," ("delimiter (\\t)")) -> ("error out"=w360:errorcluster)  [unwired: 9 in, 1 out]
            n120 = call "ATM Messages (SubVI).vi"("Message Type"=Messages."Session Terminate Message", "error in (no error)"=w360) -> ("error out"=w373:errorcluster, "Message out"=w375:string)  [unwired: 8 in]
          }
        }
        "ATM Messages" <- w22
        "Left Menu" <- w19
        "Right Menu" <- w18
        n121 = Equal?(x=w28, y=ATMStates."Stop" ("States")) -> (x = y?=w30:bool)
        n122 = Wait (ms)(milliseconds to wait=u32 50) -> ()  [unwired: 1 out]
      }
    }
    frame Error {
      # "do nothing"
    }
  }
  "error out" <- w1
  n123 = call <vilib>:"General Error Handler.vi"("error in (no error)"=w1) -> ()  [unwired: 10 in, 5 out]
